vi "NI-RFSG_Close.vi"(8 "error in":errorcluster {"code" format="%.0x"}, 11 "Handle":variant) -> (0 "error out":errorcluster {"code" format="%.0x"})   [LabVIEW 2015]
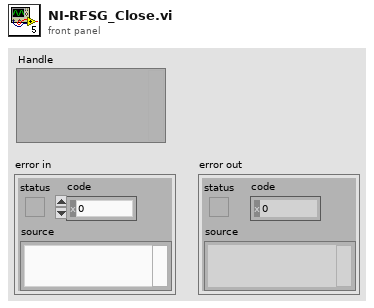
[diagram p1: front panel]
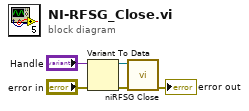
[diagram p0: block diagram]
diagram:
  n1 = Variant To Data(error in="error in", Variant="Handle") -> (data=w3:refnum<k15>, error out=w1:errorcluster)  [unwired: 1 in]
  n2 = call <instrlib>:"niRFSG Close.vi"("instrument handle"=w3, "error in"=w1) -> ("error out"=→"error out":errorcluster)  [unwired: 13 in]
